vi "Configure Output Impedance.vi"(6 "Customized Impedance (50.0 Ohm)":dbl=50.0 format="%#.2g", 8 "error in (no error)":errorcluster, 9 "Impedance (0: 50 Ohm)":u16(ring) items=["50 Ohm", "High Impedance", "Customized"], 10 "Channel (0: Channel 1)":u16(ring) items=["Channel 1", "Channel2"], 11 "VISA resource name":refnum<visa-resource-name>) -> (0 "error out":errorcluster, 3 "VISA resource name out":refnum<visa-resource-name>)   [LabVIEW 2015, in "Tektronix AFG 3000 Series.lvlib"]
doc: "Configures the output impedance for the function generator."
uses:
  Tektronix AFG 3000 Series.lvlib
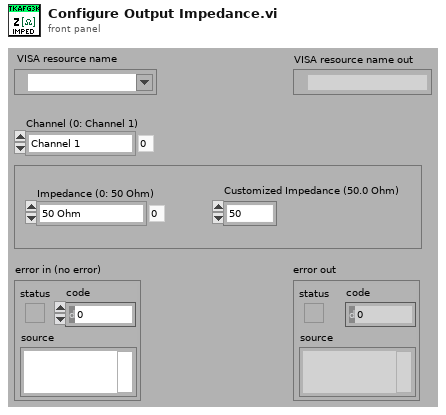
[diagram p1: front panel]
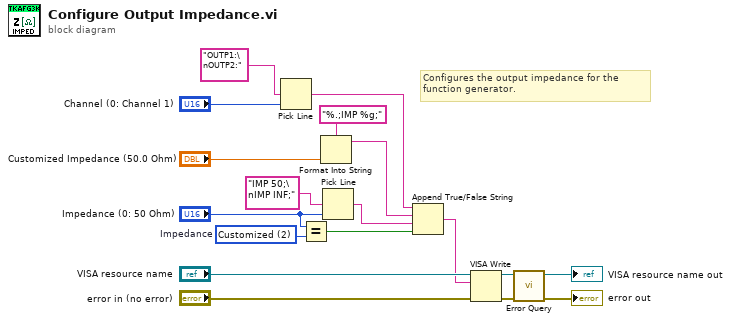
[diagram p0: block diagram]
diagram:
  w9 = u16 2 items=["50 Ohm", "High Impedance", "Customized"]  # Impedance
  # "Configures the output impedance for the \nfunction generator."
  n1 = Pick Line(multi-line string="OUTP1:\nOUTP2:" ("string (\"\")"), line index="Channel (0: Channel 1)") -> (output string=w4:string)  [unwired: 1 in]
  n2 = Equal?(x="Impedance (0: 50 Ohm)", y=w9) -> (x = y?=w7:bool)
  n3 = Format Into String(format string="%.;IMP %g;", "Customized Impedance (50.0 Ohm)") -> (resulting string=w1:string)  [unwired: 2 in, 1 out]
  n4 = Pick Line(multi-line string="IMP 50;\nIMP INF;" ("Impedance Command"), line index="Impedance (0: 50 Ohm)") -> (output string=w6:string)  [unwired: 1 in]
  n5 = Append True/False String(1:w7, 2:w6, 3:w1, 4:w4) -> (0:w5:string)
  n6 = VISA Write(VISA resource name="VISA resource name", write buffer=w5, error in (no error)="error in (no error)") -> (VISA resource name out=w14:refnum<visa-resource-name>, error out=w13:errorcluster)  [unwired: 1 out]
  n7 = call "Error Query.vi"("error in (no error)"=w13, "VISA resource name"=w14) -> ("error out"=→"error out":errorcluster, "VISA resource name out"=→"VISA resource name out":refnum<visa-resource-name>)  [unwired: 6 in, 2 out]
